vi "PathPlanner_Path_Test.vi"(8 "error in (no error)":errorcluster) -> (0 "error out":errorcluster, 3 "All Passed":bool)   [LabVIEW 2019]
uses:
  <vilib>/Rock Robotics/WPI/ThirdParty/MJansen/PathPlanner/TypeDef/PathPlannerPath.ctl
  <vilib>/Rock Robotics/WPI/ThirdParty/JAS_Junk/TrajLib/TypeDef/TRANSLATION2D.ctl
  <vilib>/Rock Robotics/WPI/ThirdParty/JAS_Junk/TrajLib/TypeDef/ROTATION2D.ctl
  <vilib>/Rock Robotics/WPI/ThirdParty/MJansen/PathPlanner/TypeDef/PathPlannerRotationTarget.ctl
  <vilib>/Rock Robotics/WPI/ThirdParty/MJansen/PathPlanner/TypeDef/PathPlannerConstraintsZone.ctl
  <vilib>/Rock Robotics/WPI/ThirdParty/MJansen/PathPlanner/TypeDef/PathPlannerPathConstraints.ctl
  <vilib>/Rock Robotics/WPI/ThirdParty/MJansen/PathPlanner/TypeDef/PathPlannerEventMarker.ctl
  <vilib>/Rock Robotics/WPI/ThirdParty/MJansen/PathPlanner/TypeDef/PathPlannerCommand.ctl
  <vilib>/Rock Robotics/WPI/ThirdParty/MJansen/PathPlanner/TypeDef/PathPlannerGoalEndState.ctl
  <vilib>/Rock Robotics/WPI/ThirdParty/MJansen/PathPlanner/TypeDef/PathPlannerPathPoint.ctl
  <vilib>/Rock Robotics/WPI/ThirdParty/JAS_Junk/TrajLib/Conv_Deg_Radians.vi
  <vilib>/Rock Robotics/WPI/ThirdParty/JAS_Junk/TrajLib/Rotation2d_CreateAngle.vi
  <vilib>/Rock Robotics/WPI/ThirdParty/JAS_Junk/TrajLib/Pose2d_New_TRRO.vi
  <vilib>/Rock Robotics/WPI/ThirdParty/MJansen/PathPlanner/VI/PathPlanner_Path_GetPoint.vi
  <vilib>/Rock Robotics/WPI/ThirdParty/MJansen/PathPlanner/VI/PathPlanner_PathPoint_GetAll.vi
  <vilib>/Rock Robotics/WPI/ThirdParty/JAS_Junk/TrajLib/Translation2d_Minus.vi
  <vilib>/Rock Robotics/WPI/ThirdParty/JAS_Junk/TrajLib/Translation2d_GetAngle.vi
  <vilib>/Rock Robotics/WPI/ThirdParty/MJansen/PathPlanner/VI/PathPlanner_Path_IsReversed.vi
  <vilib>/Rock Robotics/WPI/ThirdParty/JAS_Junk/TrajLib/Rotation2d_GetDegrees.vi
  <vilib>/Rock Robotics/WPI/ThirdParty/JAS_Junk/TrajLib/MathUtil_InputModulus.vi
  <vilib>/Rock Robotics/WPI/ThirdParty/JAS_Junk/TrajLib/Translation2d_GetXY.vi
  <vilib>/Rock Robotics/WPI/ThirdParty/JAS_Junk/TrajLib/Rotation2d_CreateXY.vi
  <vilib>/Rock Robotics/WPI/ThirdParty/JAS_Junk/TrajLib/Rotation2d_GetRadians.vi
  <vilib>/Rock Robotics/WPI/ThirdParty/JAS_Junk/TrajLib/Util_CalcDist.vi
  <vilib>/Rock Robotics/WPI/ThirdParty/JAS_Junk/TrajLib/Trajectory_Library.lvlib
  <vilib>/Rock Robotics/WPI/ThirdParty/MJansen/PathPlanner/PathPlanner24.lvlib
panel:
  out "PathPlannerPath 2":T1={"BezierPoints"=[], "PreviewStartingRotation"={"VALUE"=0.0, "COS"=1.0, "SIN"=0.0}, "Reversed"=FALSE, "RotationTargets"=[], "ConstraintZones"=[], "EventMarkers"=[], "GlobalConstraints"={"MaxVelocityMps;"=0.0, "MaxAccelerationMpsSq;"=0.0, "MaxAngularVelRadPsEc;"=0.0, "MaxAngularAccRadPSecSq"=0.0, "Exists"=FALSE}, "GoalEndState"={"Velocity"=0.0, "Rotation"={"VALUE"=0.0, "COS"=1.0, "SIN"=0.0}}, "AllPoints"=[]} {"AllPoints"."HolonomicRotation"."SIN" format="%13.4f"; "AllPoints"."HolonomicRotation"."COS" format="%13.4f"; "AllPoints"."HolonomicRotation"."VALUE" format="%13.4f"; "AllPoints"."Position"."Y" format="%14.3f"; "AllPoints"."Position"."X" format="%14.3f"; "GoalEndState"."Rotation"."SIN" format="%13.4f"; "GoalEndState"."Rotation"."COS" format="%13.4f"; "GoalEndState"."Rotation"."VALUE" format="%13.4f"; "EventMarkers"."lastRobotPos"."Y" format="%14.3f"; "EventMarkers"."lastRobotPos"."X" format="%14.3f"; "EventMarkers"."markerPos"."Y" format="%14.3f"; "EventMarkers"."markerPos"."X" format="%14.3f"; "RotationTargets"."target"."SIN" format="%13.4f"; "RotationTargets"."target"."COS" format="%13.4f"; "RotationTargets"."target"."VALUE" format="%13.4f"; "PreviewStartingRotation"."SIN" format="%13.4f"; "PreviewStartingRotation"."COS" format="%13.4f"; "PreviewStartingRotation"."VALUE" format="%13.4f"; "BezierPoints"."Y" format="%14.3f"; "BezierPoints"."X" format="%14.3f"}
  out "Error 2":bool
  out "PathPlannerPath":T1={"BezierPoints"=[], "PreviewStartingRotation"={"VALUE"=0.0, "COS"=1.0, "SIN"=0.0}, "Reversed"=FALSE, "RotationTargets"=[], "ConstraintZones"=[], "EventMarkers"=[], "GlobalConstraints"={"MaxVelocityMps;"=0.0, "MaxAccelerationMpsSq;"=0.0, "MaxAngularVelRadPsEc;"=0.0, "MaxAngularAccRadPSecSq"=0.0, "Exists"=FALSE}, "GoalEndState"={"Velocity"=0.0, "Rotation"={"VALUE"=0.0, "COS"=1.0, "SIN"=0.0}}, "AllPoints"=[]} {"AllPoints"."HolonomicRotation"."SIN" format="%13.4f"; "AllPoints"."HolonomicRotation"."COS" format="%13.4f"; "AllPoints"."HolonomicRotation"."VALUE" format="%13.4f"; "AllPoints"."Position"."Y" format="%14.3f"; "AllPoints"."Position"."X" format="%14.3f"; "GoalEndState"."Rotation"."SIN" format="%13.4f"; "GoalEndState"."Rotation"."COS" format="%13.4f"; "GoalEndState"."Rotation"."VALUE" format="%13.4f"; "EventMarkers"."lastRobotPos"."Y" format="%14.3f"; "EventMarkers"."lastRobotPos"."X" format="%14.3f"; "EventMarkers"."markerPos"."Y" format="%14.3f"; "EventMarkers"."markerPos"."X" format="%14.3f"; "RotationTargets"."target"."SIN" format="%13.4f"; "RotationTargets"."target"."COS" format="%13.4f"; "RotationTargets"."target"."VALUE" format="%13.4f"; "PreviewStartingRotation"."SIN" format="%13.4f"; "PreviewStartingRotation"."COS" format="%13.4f"; "PreviewStartingRotation"."VALUE" format="%13.4f"; "BezierPoints"."Y" format="%14.3f"; "BezierPoints"."X" format="%14.3f"}
  out "Error":bool
  out "Passed 3":bool
  out "Passed 2":bool
  out "Passed 1":bool
  # "DifferentialStartingPose"
  # "HolomonicStartingPoseSet"
  # "HolomonicStartingPose Null"
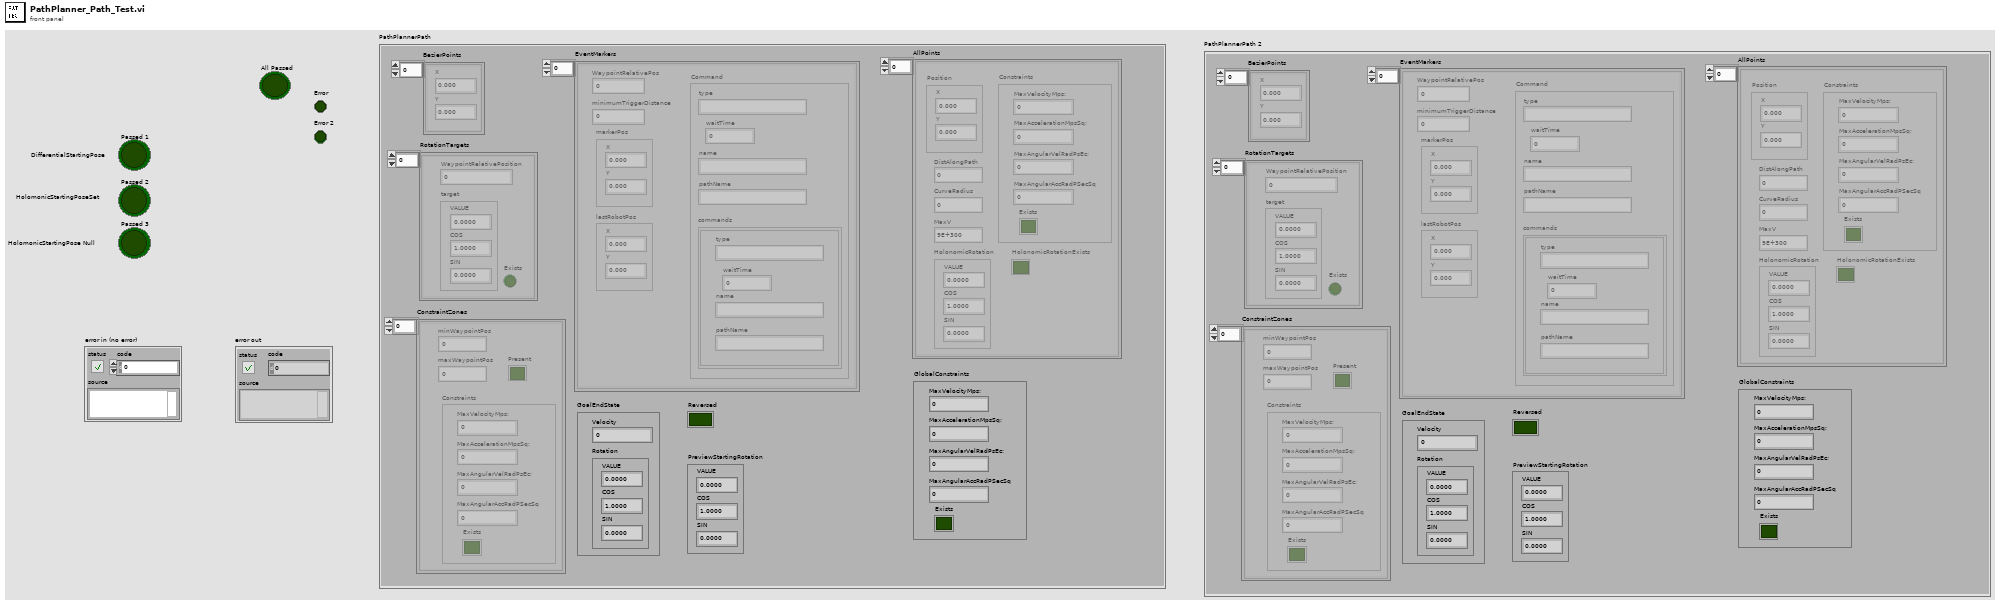
[diagram p1: front panel]
types:
  T1 = typedef "PathPlanner24.lvlib/PathPlannerPath.ctl" = cluster{"BezierPoints":T2[], "PreviewStartingRotation":T3, "Reversed":bool, "RotationTargets":T4[], "ConstraintZones":T5[], "EventMarkers":T7[], "GlobalConstraints":T6, "GoalEndState":T9, "AllPoints":T10[]}
  T2 = typedef "Trajectory_Library.lvlib/TRANSLATION2D.ctl" = cluster{"X":dbl, "Y":dbl}
  T3 = typedef "Trajectory_Library.lvlib/ROTATION2D.ctl" = cluster{"VALUE":dbl, "COS":dbl, "SIN":dbl}
  T4 = typedef "PathPlanner24.lvlib/PathPlannerRotationTarget.ctl" = cluster{"target":T3, "WaypointRelativePosition":dbl, "Exists":bool}
  T5 = typedef "PathPlanner24.lvlib/PathPlannerConstraintsZone.ctl" = cluster{"minWaypointPos":dbl, "maxWaypointPos":dbl, "Constraints":T6, "Present":bool}
  T6 = typedef "PathPlanner24.lvlib/PathPlannerPathConstraints.ctl" = cluster{"MaxVelocityMps;":dbl, "MaxAccelerationMpsSq;":dbl, "MaxAngularVelRadPsEc;":dbl, "MaxAngularAccRadPSecSq":dbl, "Exists":bool}
  T7 = typedef "PathPlanner24.lvlib/PathPlannerEventMarker.ctl" = cluster{"WaypointRelativePos":dbl, "minimumTriggerDistance":dbl, "markerPos":T2, "lastRobotPos":T2, "Command":T8}
  T8 = typedef "PathPlanner24.lvlib/PathPlannerCommand.ctl" = cluster{"waitTime":dbl, "name":string, "type":string, "pathName":string, "commands":cluster{"type":string, "waitTime":dbl, "name":string, "pathName":string}[]}
  T9 = typedef "PathPlanner24.lvlib/PathPlannerGoalEndState.ctl" = cluster{"Velocity":dbl, "Rotation":T3}
  T10 = typedef "PathPlanner24.lvlib/PathPlannerPathPoint.ctl" = cluster{"Position":T2, "HolonomicRotation":T3, "DistAlongPath":dbl, "CurveRadius":dbl, "MaxV":dbl, "Constraints":T6, "HolonomicRotationExists":bool}
  T11 = typedef "Trajectory_Library.lvlib/POSE2D.ctl" = cluster{"TRANSLATION":T2, "ROTATION":T3}
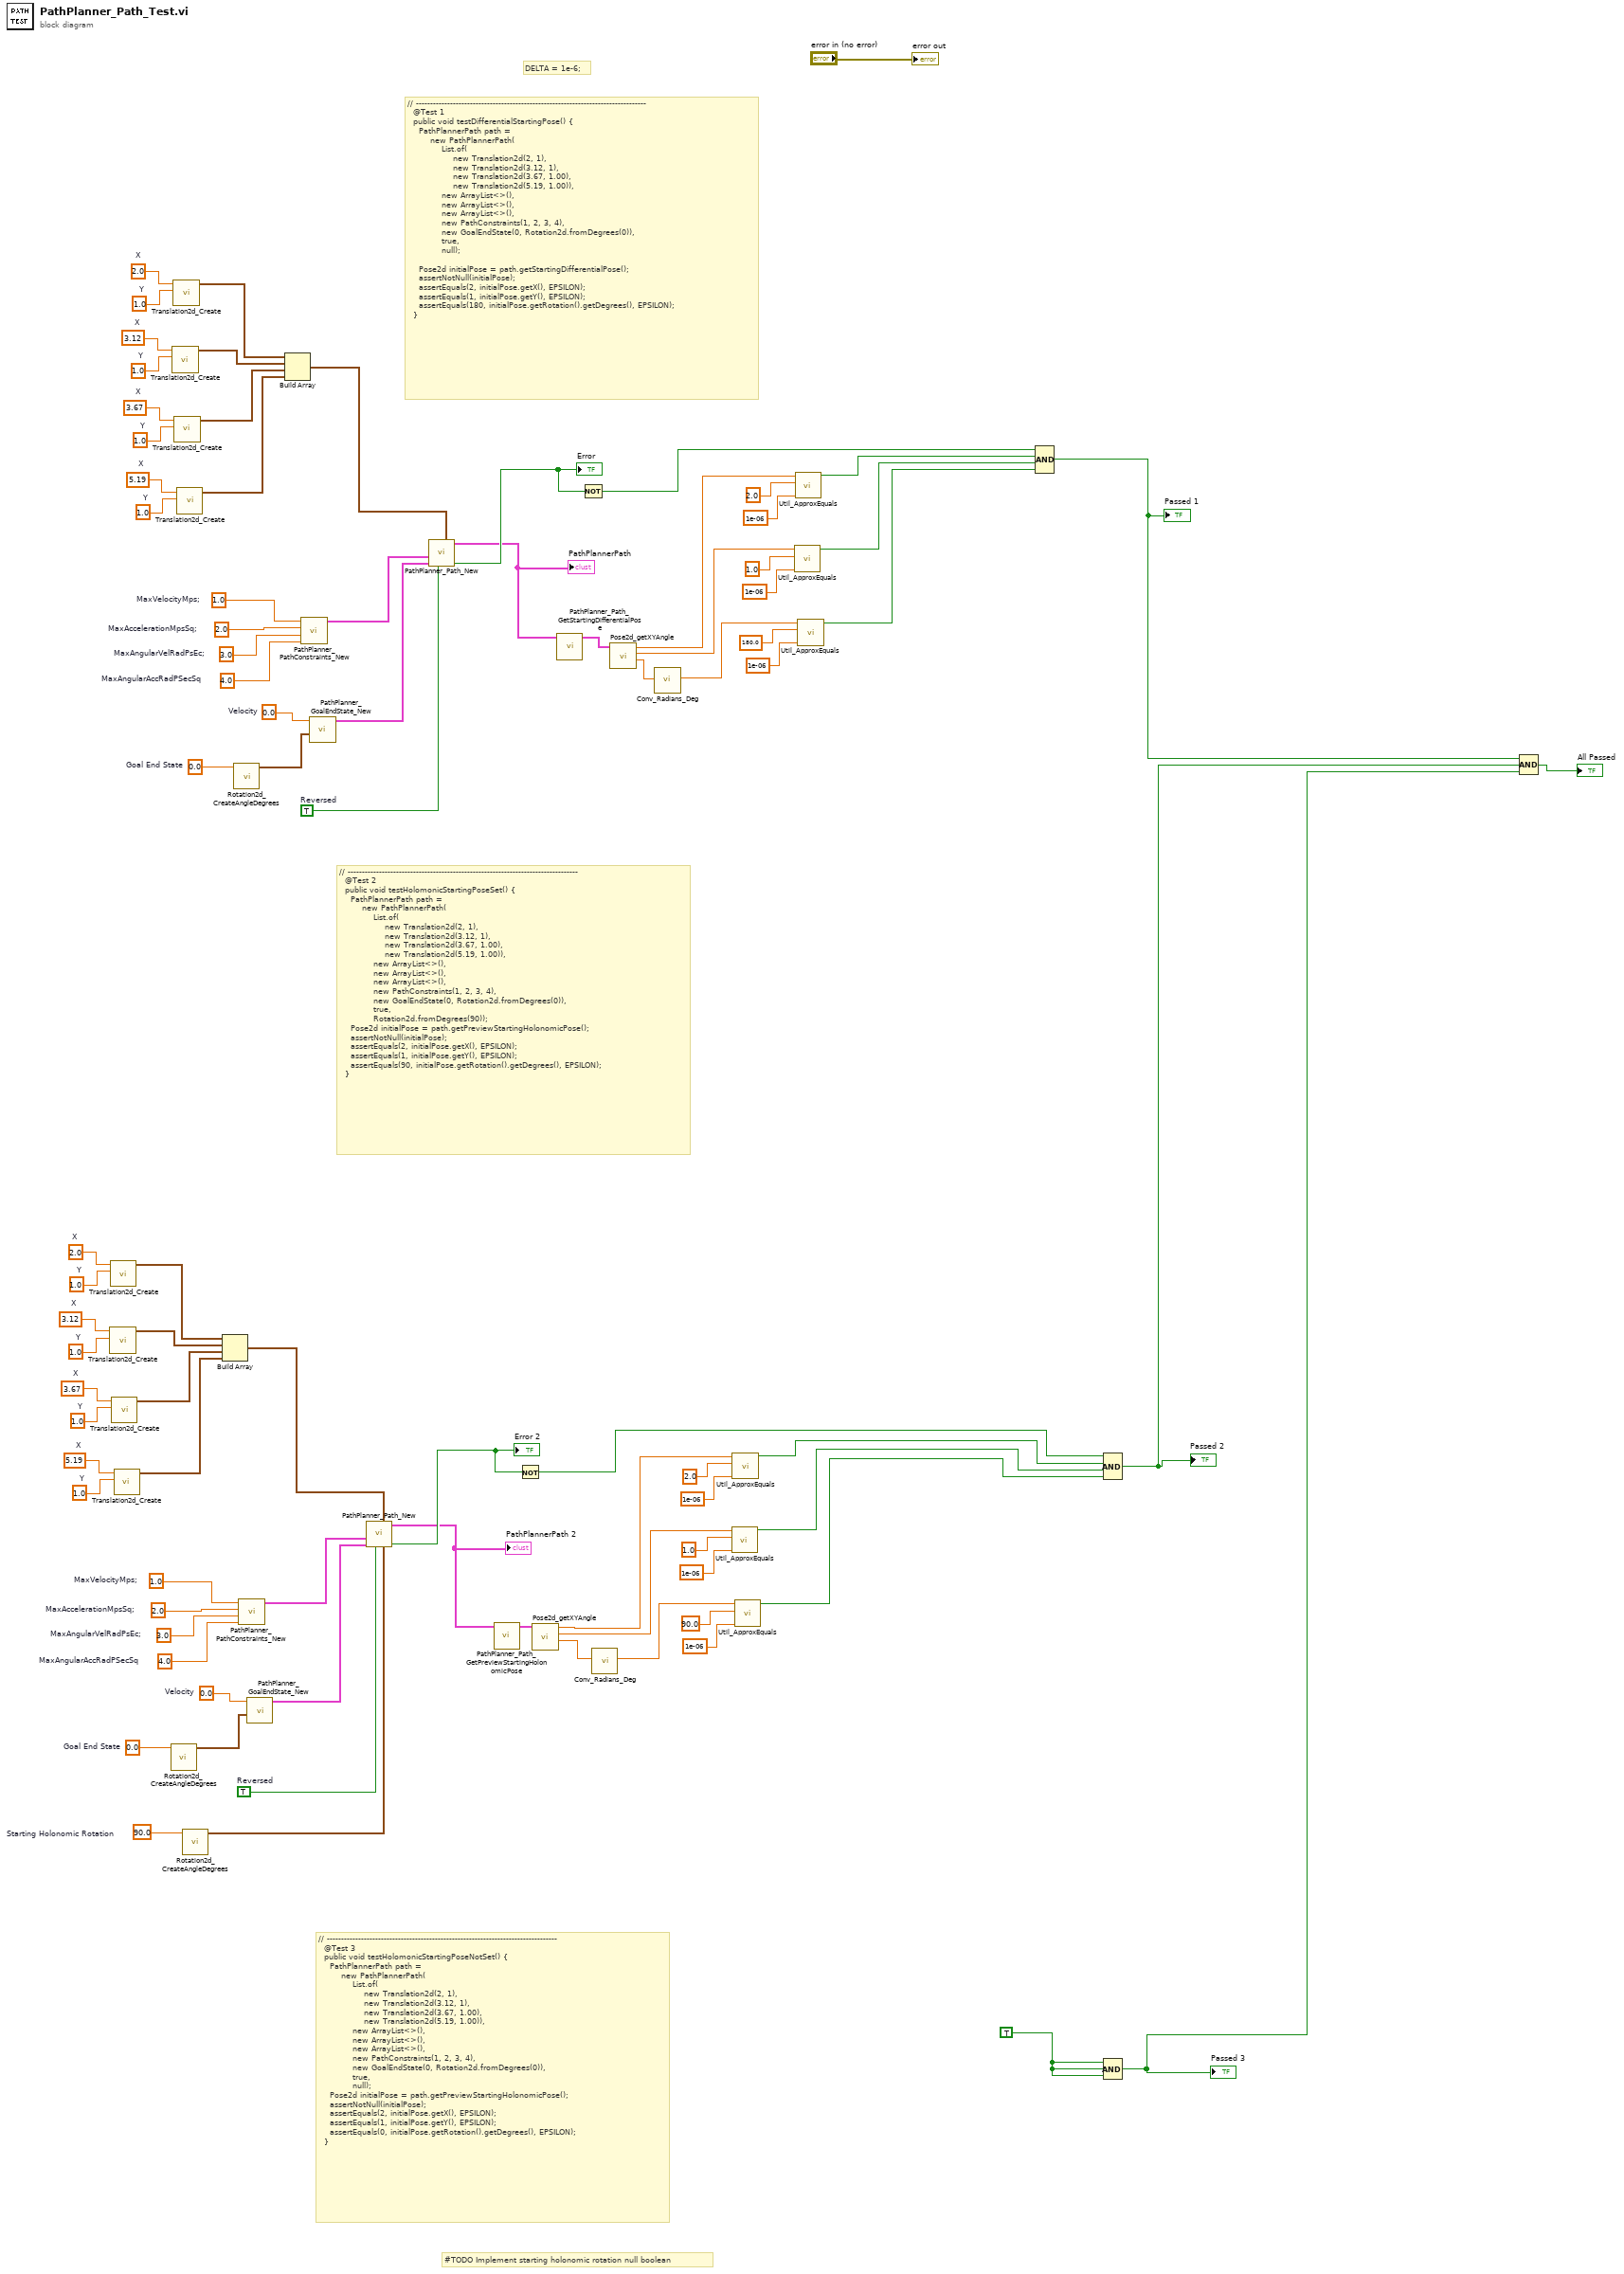
[diagram p0: block diagram]
diagram:
  w1 = TRUE
  w12 = 90.0  # Starting Holonomic Rotation
  w18 = 0.0  # Velocity
  w20 = 0.0  # Goal End State
  w21 = TRUE  # Reversed
  w28 = 5.19  # X
  w27 = 1.0  # Y
  w30 = 2.0  # X
  w29 = 1.0  # Y
  w32 = 3.67  # X
  w31 = 1.0  # Y
  w34 = 3.12  # X
  w33 = 1.0  # Y
  w40 = 1.0  # MaxVelocityMps;
  w41 = 2.0  # MaxAccelerationMpsSq;
  w42 = 3.0  # MaxAngularVelRadPsEc;
  w43 = 4.0  # MaxAngularAccRadPSecSq
  w56 = 0.0  # Velocity
  w58 = 0.0  # Goal End State
  w59 = TRUE  # Reversed
  w66 = 5.19  # X
  w65 = 1.0  # Y
  w68 = 2.0  # X
  w67 = 1.0  # Y
  w70 = 3.67  # X
  w69 = 1.0  # Y
  w72 = 3.12  # X
  w71 = 1.0  # Y
  w79 = 1.0  # MaxVelocityMps;
  w80 = 2.0  # MaxAccelerationMpsSq;
  w81 = 3.0  # MaxAngularVelRadPsEc;
  w82 = 4.0  # MaxAngularAccRadPSecSq
  # "#TODO Implement starting holonomic rotation null boolean"
  # "// ---------------------------------------------------------------------------------\n  @Test 3\n  public void testHolomonicStartingPoseNotSet() {\n    PathPlannerPath path =\n        new PathPlannerPath(\n            List.of(\n                new Translation2d(2, 1),\n                new Translation2d(3.12, 1),\n                new Translation2d(3.67, 1.00),\n                new Translation2d(5.19, 1.00)),\n            new ArrayList<>(),\n            new ArrayList<>(),\n            new ArrayList<>(),\n            new PathConstraints(1, 2, 3, 4),\n            new GoalEndState(0, Rotation2d.fromDegrees(0)),\n            true,\n            null);\n    Pose2d initialPose = path.getPreviewStartingHolonomicPose();\n    assertNotNull(initialPose);\n    assertEquals(2, initialPose.getX(), EPSILON);\n    assertEquals(1, initialPose.getY(), EPSILON);\n    assertEquals(0, initialPose.getRotation().getDegrees(), EPSILON);\n  }"
  # "// ---------------------------------------------------------------------------------\n  @Test 2\n  public void testHolomonicStartingPoseSet() {\n    PathPlannerPath path =\n        new PathPlannerPath(\n            List.of(\n                new Translation2d(2, 1),\n                new Translation2d(3.12, 1),\n                new Translation2d(3.67, 1.00),\n                new Translation2d(5.19, 1.00)),\n            new ArrayList<>(),\n            new ArrayList<>(),\n            new ArrayList<>(),\n            new PathConstraints(1, 2, 3, 4),\n            new GoalEndState(0, Rotation2d.fromDegrees(0)),\n            true,\n            Rotation2d.fromDegrees(90));\n    Pose2d initialPose = path.getPreviewStartingHolonomicPose();\n    assertNotNull(initialPose);\n    assertEquals(2, initialPose.getX(), EPSILON);\n    assertEquals(1, initialPose.getY(), EPSILON);\n    assertEquals(90, initialPose.getRotation().getDegrees(), EPSILON);\n  }"
  # "// ---------------------------------------------------------------------------------\n  @Test 1\n  public void testDifferentialStartingPose() {\n    PathPlannerPath path =\n        new PathPlannerPath(\n            List.of(\n                new Translation2d(2, 1),\n                new Translation2d(3.12, 1),\n                new Translation2d(3.67, 1.00),\n                new Translation2d(5.19, 1.00)),\n            new ArrayList<>(),\n            new ArrayList<>(),\n            new ArrayList<>(),\n            new PathConstraints(1, 2, 3, 4),\n            new GoalEndState(0, Rotation2d.fromDegrees(0)),\n            true,\n            null);\n\n    Pose2d initialPose = path.getStartingDifferentialPose();\n    assertNotNull(initialPose);\n    assertEquals(2, initialPose.getX(), EPSILON);\n    assertEquals(1, initialPose.getY(), EPSILON);\n    assertEquals(180, initialPose.getRotation().getDegrees(), EPSILON);\n  }"
  # "DELTA = 1e-6;"
  n1 = call <vilib>:"Translation2d_Create.vi"("Y"=w33, "X"=w34) -> ("TRANSLATION"=w25:T2)  [unwired: 9 in]
  n2 = call <vilib>:"Translation2d_Create.vi"("Y"=w29, "X"=w30) -> ("TRANSLATION"=w26:T2)  [unwired: 9 in]
  n3 = call <vilib>:"Translation2d_Create.vi"("Y"=w31, "X"=w32) -> ("TRANSLATION"=w24:T2)  [unwired: 9 in]
  n4 = call <vilib>:"Translation2d_Create.vi"("Y"=w27, "X"=w28) -> ("TRANSLATION"=w23:T2)  [unwired: 9 in]
  n5 = call <vilib>:"Rotation2d_CreateAngleDegrees.vi"("Angle_Degrees"=w20) -> ("ROTATION"=w19:T3)  [unwired: 10 in]
  n6 = call <vilib>:"Translation2d_Create.vi"("Y"=w71, "X"=w72) -> ("TRANSLATION"=w63:T2)  [unwired: 9 in]
  n7 = call <vilib>:"Translation2d_Create.vi"("Y"=w67, "X"=w68) -> ("TRANSLATION"=w64:T2)  [unwired: 9 in]
  n8 = call <vilib>:"Translation2d_Create.vi"("Y"=w69, "X"=w70) -> ("TRANSLATION"=w62:T2)  [unwired: 9 in]
  n9 = call <vilib>:"Translation2d_Create.vi"("Y"=w65, "X"=w66) -> ("TRANSLATION"=w61:T2)  [unwired: 9 in]
  n10 = call <vilib>:"Rotation2d_CreateAngleDegrees.vi"("Angle_Degrees"=w12) -> ("ROTATION"=w11:T3)  [unwired: 10 in]
  n11 = Build Array(w26, w25, w24, w23) -> (w22:T2[])
  n12 = call <vilib>:"Rotation2d_CreateAngleDegrees.vi"("Angle_Degrees"=w58) -> ("ROTATION"=w57:T3)  [unwired: 10 in]
  n13 = call <vilib>:"PathPlanner_PathConstraints_New.vi"("MaxAngularAccRadPSecSq"=w43, "MaxAngularVelRadPsEc;"=w42, "MaxAccelerationMpsSq;"=w41, "MaxVelocityMps;"=w40) -> ("PathPlannerConstraints"=w35:T6)  [unwired: 7 in]
  n14 = call <vilib>:"PathPlanner_GoalEndState_New.vi"("Rotation"=w19, "Velocity"=w18) -> ("GoalEndState"=w17:T9)  [unwired: 9 in]
  n15 = Build Array(w64, w63, w62, w61) -> (w60:T2[])
  n16 = call <vilib>:"PathPlanner_PathConstraints_New.vi"("MaxAngularAccRadPSecSq"=w82, "MaxAngularVelRadPsEc;"=w81, "MaxAccelerationMpsSq;"=w80, "MaxVelocityMps;"=w79) -> ("PathPlannerConstraints"=w73:T6)  [unwired: 7 in]
  n17 = call <vilib>:"PathPlanner_GoalEndState_New.vi"("Rotation"=w57, "Velocity"=w56) -> ("GoalEndState"=w55:T9)  [unwired: 9 in]
  n18 = call <vilib>:"PathPlanner_Path_New.vi"("PreviewStartingRotation"=w11, "BezierPoints"=w22, "Reversed"=w21, "GoalEndState"=w17, "GlobalConstraints"=w35) -> ("Error"=w16:bool, "PathPlannerPath"=w10:T1)  [unwired: 5 in]
  "Error 2" <- w16
  "PathPlannerPath 2" <- w10
  n19 = call <vilib>:"PathPlanner_Path_New.vi"("BezierPoints"=w60, "Reversed"=w59, "GoalEndState"=w55, "GlobalConstraints"=w73) -> ("Error"=w54:bool, "PathPlannerPath"=w52:T1)  [unwired: 6 in]
  "Error" <- w54
  "PathPlannerPath" <- w52
  n20 = call <vilib>:"PathPlanner_Path_GetPreviewStartingHolonomicPose.vi"("PathPlannerPath"=w10) -> ("PreviewStartingPose"=w9:T11)  [unwired: 10 in]
  n21 = Not(x=w16) -> (.not. x?=w5:bool)
  n22 = call <vilib>:"Pose2d_getXYAngle.vi"("in POSE"=w9) -> ("Angle"=w6:dbl, "Y"=w7:dbl, "X"=w8:dbl)  [unwired: 8 in]
  n23 = call <vilib>:"PathPlanner_Path_GetStartingDifferentialPose.vi"("PathPlannerPath"=w52) -> ("StartingDifferentialPose"=w51:T11)  [unwired: 10 in]
  n24 = Not(x=w54) -> (.not. x?=w53:bool)
  n25 = call <vilib>:"Conv_Radians_Deg.vi"("Radians"=w6) -> ("Degrees"=w13:dbl)  [unwired: 10 in]
  n26 = call <vilib>:"Pose2d_getXYAngle.vi"("in POSE"=w51) -> ("Angle"=w50:dbl, "Y"=w48:dbl, "X"=w49:dbl)  [unwired: 8 in]
  n27 = call <vilib>:"Conv_Radians_Deg.vi"("Radians"=w50) -> ("Degrees"=w45:dbl)  [unwired: 10 in]
  n28 = call <vilib>:"Util_ApproxEquals.vi"("Tolerance"=1e-06, "Value 2"=1.0, "Value 1"=w7) -> ("ApproxEquals"=w3:bool)  [unwired: 8 in]
  n29 = call <vilib>:"Util_ApproxEquals.vi"("Tolerance"=1e-06, "Value 2"=2.0, "Value 1"=w8) -> ("ApproxEquals"=w4:bool)  [unwired: 8 in]
  n30 = call <vilib>:"Util_ApproxEquals.vi"("Tolerance"=1e-06, "Value 2"=90.0, "Value 1"=w13) -> ("ApproxEquals"=w2:bool)  [unwired: 8 in]
  n31 = call <vilib>:"Util_ApproxEquals.vi"("Tolerance"=1e-06, "Value 2"=1.0, "Value 1"=w48) -> ("ApproxEquals"=w74:bool)  [unwired: 8 in]
  n32 = call <vilib>:"Util_ApproxEquals.vi"("Tolerance"=1e-06, "Value 2"=2.0, "Value 1"=w49) -> ("ApproxEquals"=w86:bool)  [unwired: 8 in]
  n33 = call <vilib>:"Util_ApproxEquals.vi"("Tolerance"=1e-06, "Value 2"=180.0, "Value 1"=w45) -> ("ApproxEquals"=w44:bool)  [unwired: 8 in]
  n34 = Compound Arithmetic op=AND(w53, w86, w74, w44) -> (w85:bool)
  "Passed 1" <- w85
  n35 = Compound Arithmetic op=AND(w5, w4, w3, w2) -> (w84:bool)
  "Passed 2" <- w84
  n36 = Compound Arithmetic op=AND(w1, w1, w1) -> (w83:bool)
  "Passed 3" <- w83
  n37 = Compound Arithmetic op=AND(w85, w84, w83) -> (→"All Passed":bool)
  "error out" <- "error in (no error)"
